vi "Toggle with previous input control.vi"(1 "Control":bool, 2 "Previous Input":T1=enum."Forward", 3 "Reset to Previous Input?":bool) -> (0 "Output":T1=enum."Forward")   [LabVIEW 2014]
uses:
  <vilib>/Rock Robotics/WPI/Solenoid/WPI_SolenoidValue.ctl
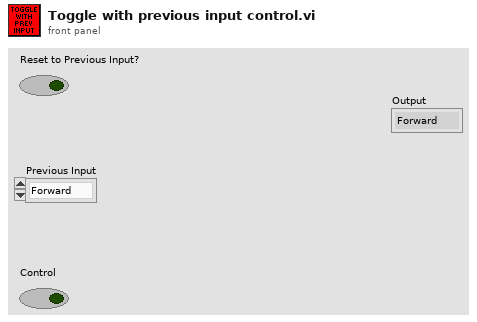
[diagram p1: front panel]
types:
  T1 = typedef "WPI_SolenoidValue.ctl" = enum16{"Off", "On", "Forward", "Reverse"}
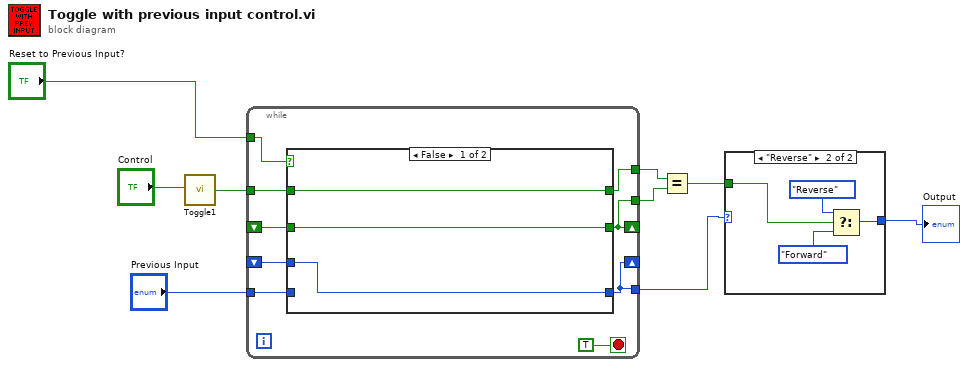
[diagram p0: block diagram]
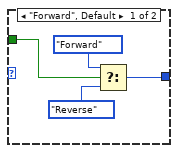
[diagram p2: hidden frame]
diagram:
  n1 = call "Toggle1.vi"("Boolean"="Control") -> ("Driver Switch 2"=w1:bool)
  n2 = while {
    tunnel: w1 -> [w14]
    tunnel: "Reset to Previous Input?" -> [w17]
    tunnel: "Previous Input" -> [w16]
    shift-right: [w12] -> _
    shift-left: _ -> [w15]
    shift-right: [w11] -> _
    shift-left: _ -> [w13]
    tunnel: [w12] -> w4
    tunnel: [w11] -> w5
    tunnel: [w10] -> w6
    stop <- TRUE stop-if-true
    n3 = case shown="False" w17 {
      tunnel: w16 -> [_ w23]
      tunnel: [w21 w23] -> w12
      tunnel: w15 -> [w21 _]
      tunnel: w14 -> [w19 w22]
      tunnel: [w20 w22] -> w11
      tunnel: w13 -> [w20 _]
      tunnel: [w19 w22] -> w10
      frame False {
      }
      frame True {
      }
    }
  }
  n4 = Equal?(x=w6, y=w5) -> (x = y?=w3:bool)
  n5 = case shown="\"Reverse\"" w4 {
    tunnel: w3 -> [w27 w28]
    tunnel: [w26 w29] -> w2
    frame "Forward", Default {
      n6 = Select(t=WPI_SolenoidValue."Forward" ("Output"), s=w27, f=WPI_SolenoidValue."Reverse" ("Output")) -> (s? t:f=w26:T1)
    }
    frame "Reverse" {
      n7 = Select(t=WPI_SolenoidValue."Reverse" ("Output"), s=w28, f=WPI_SolenoidValue."Forward" ("Output")) -> (s? t:f=w29:T1)
    }
  }
  "Output" <- w2
